vi "Write menu object names.vi"(8 "error in (no error)":errorcluster, 10 "Menu object names":string[](array[string]), 11 "Menu object array in":refnum<class "Menu object array.lvclass">) -> (0 "error out":errorcluster, 3 "Menu object array out":refnum<class "Menu object array.lvclass">)   [LabVIEW 2015, in "Menu object array.lvclass"]
uses:
  Menu object array.lvclass
  Menu object array.lvclass/Menu object array.ctl
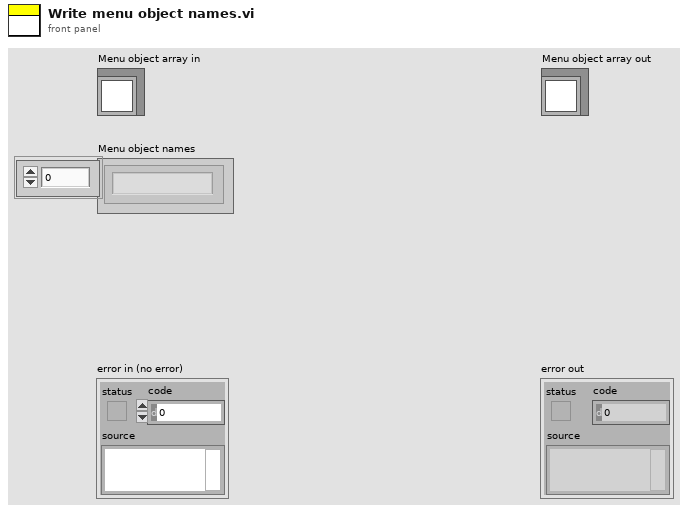
[diagram p1: front panel]
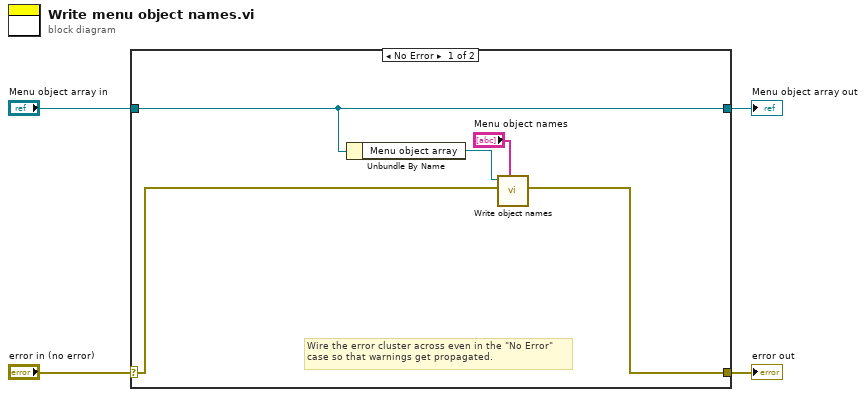
[diagram p0: block diagram]
diagram:
  n1 = case shown="No Error" "error in (no error)" {
    selector: "error in (no error)" -> [w6 w11]
    tunnel: [w5 w11] -> w3
    tunnel: [w9 w10] -> w1
    tunnel: "Menu object array in" -> [w9 w10]
    frame No Error {
      # "Wire the error cluster across even in the \"No Error\"\ncase so that warnings get propagated."
      n2 = Unbundle By Name(w9) -> ("Menu object array"=w8:refnum<vi>)
      n3 = call "Write object names.vi"("Object names"="Menu object names", "Error In"=w6, "Menu object array ref"=w8) -> ("Error Out"=w5:errorcluster)  [unwired: 8 in]
    }
    frame Error {
    }
  }
  "error out" <- w3
  "Menu object array out" <- w1
